vi "CRYLimits.vi"(0 "Setup in":T1={"No.VI"=0, "Category"="", "StepName"="", "Seq setup flattened"="", "Comment"="", "Steps config."=[], "Jump config"=[], "Start"=0.0, "Increment"=0.0, "Name"="Pa", "Unit"="Pa", "Y data"=1, "Y prefix"="", "Y dB ref"=1.0, "Y unit"="", "Repeat State Array"=[]} {"Repeat State Array"."Start" format="%#_5g"; "Y dB ref" format="%.1f"; "Y data" items=["dB", "Lin"]; "Start" format="%#_5g"}, 5 "Data in":T4 {"Z data" items=["dB", "Lin"]; "X data" items=["dB", "Lin"]; "Y data" items=["dB", "Lin"]; "Z dB ref" format="%.1f"; "Z axis" items=["Log", "Lin"]; "X dB ref" format="%.1f"; "X axis" items=["Log", "Lin"]; "Y axis" items=["Log", "Lin"]; "Y dB ref" format="%.1f"; "Curve"."z" format="%.2f"; "Curve"."y" format="%.2f"; "Curve"."x" format="%.2f"}, 7 "Results In":T2[](array[typedef]) {"Margin" format="%.2f"}, 9 "Seq setup in":string, 11 "Step Name":string, 12 "Hardware in":string, 13 "Calibration in":string) -> (3 "Types Out":string[](array[string]), 4 "Inserted Names Out":string[](array[string]), 6 "Data Out":T4 {"Z data" items=["dB", "Lin"]; "X data" items=["dB", "Lin"]; "Y data" items=["dB", "Lin"]; "Z dB ref" format="%.1f"; "Z axis" items=["Log", "Lin"]; "X dB ref" format="%.1f"; "X axis" items=["Log", "Lin"]; "Y axis" items=["Log", "Lin"]; "Y dB ref" format="%.1f"; "Curve"."z" format="%.2f"; "Curve"."y" format="%.2f"; "Curve"."x" format="%.2f"}, 8 "Results Out":T2[](array[typedef]) {"Margin" format="%.2f"}, 10 "Waveforms Out":T3[](array[typedef]) {"Y dB ref" format="%.1f"; "Y axis" items=["Log", "Lin"]; "Y data" items=["dB", "Lin"]; "X data" items=["dB", "Lin"]})   [LabVIEW 2013]
uses:
  Typedef Control/CRYData Cluster Array.ctl
  Typedef Control/CRYData Cluster.ctl
  Typedef Control/CRYWaveform Cluster.ctl
  Typedef Control/CRYResult Cluster.ctl
  Typedef Control/CRYStep.ctl
  <vilib>/event_ctls.llb/eventvkey.ctl
  Task Sequence/CRYProject Run Control Global.vi
  CRYStepSetup/CRYStepSetup Global.vi
  CRYLimit edit global.vi
  CRYMainGlobal.vi
panel:
  in  "Output failed":bool
  in  "Lim Curve axis lo":u16
  in  "Lim Curve axis up":u16
  out "Name":string
  in  "stop":bool
  in  "magn/phase":u16
  out "Multi unit":string="(und)"
  out "Multi Limit":cluster{dbl, dbl}(slide)={100.0, 4.285714285714286} caption="Upper limit" scale=-7.0..2.0 scale format="%.1p"
  out "Multi value":dbl(slide) scale=-7.0..2.0 scale format="%#.3p"
  in  "Lower Limit Type":u16
  in  "Upper Limit Type":u16
  in  "X-Resolution":u8
  in  "Data Selection Lower":u16
  in  "Data Selection Upper":u16
  in  "X axis":u16(slide)=1
  in  "Type":u16(slide)=1
  out "Limits Graph":cluster{"element":cluster{"x":dbl, "y":dbl}[]}[](graph)
  out "Limits Settings":bool
  in  "single val":bool
  in  "Data":cluster{"Hz":dbl, "dB":dbl}[](array[cluster])=[{"Hz"=1000.0, "dB"=125.0}] {"dB" format="%.1f"}
  in  "Tolerance":u16(ring)=2 caption="Alignment" items=["Individual Pts.", "Absolute Limits", "Floating Limits", "Floating Data", "Aligned Limits", "Aligned Data"]
  in  "Upper Limit":cluster{"Hz":dbl, "y":dbl}[](array[cluster])=[{"Hz"=1000.0, "y"=125.0}] {"y" format="%.1f"}
  in  "Lower Limit":cluster{"Hz":dbl, "y":dbl}[](array[cluster])=[{"Hz"=1000.0, "y"=125.0}] {"y" format="%.1f"}
  out "Data Out":cluster{dbl, dbl}[](array[cluster]) {"?" format="%.2f"; "?" format="%.2f"}
  out "Upper Limit Out":cluster{dbl, dbl}[](array[cluster]) {"?" format="%.2f"; "?" format="%.2f"}
  out "Lower Limit Out":cluster{dbl, dbl}[](array[cluster]) {"?" format="%.2f"; "?" format="%.2f"}
  in  "Align Reference":cluster{dbl, dbl}={1000.0, 0.0} {"?" format="%.1f"}
  out "Verdict":bool=TRUE
  out "Align Reference Out":cluster{dbl, dbl} {"?" format="%.2f"; "?" format="%.2f"}
  in  "Limits":u16(ring)=2 items=["Upper Only", "Lower Only", "Upper & Lower"]
  in  "Y-Resolution":u8
  out "max":dbl format="%.2f"
  out "min":dbl format="%.2f"
  out "y value":dbl format="%#.3p"
  out "Margin":dbl=-inf format="%_3p"
  in  "x float":bool caption="Float Limits in X"
  out "Unit":string
  out "Curve Name":string
  in  "Manual?":bool
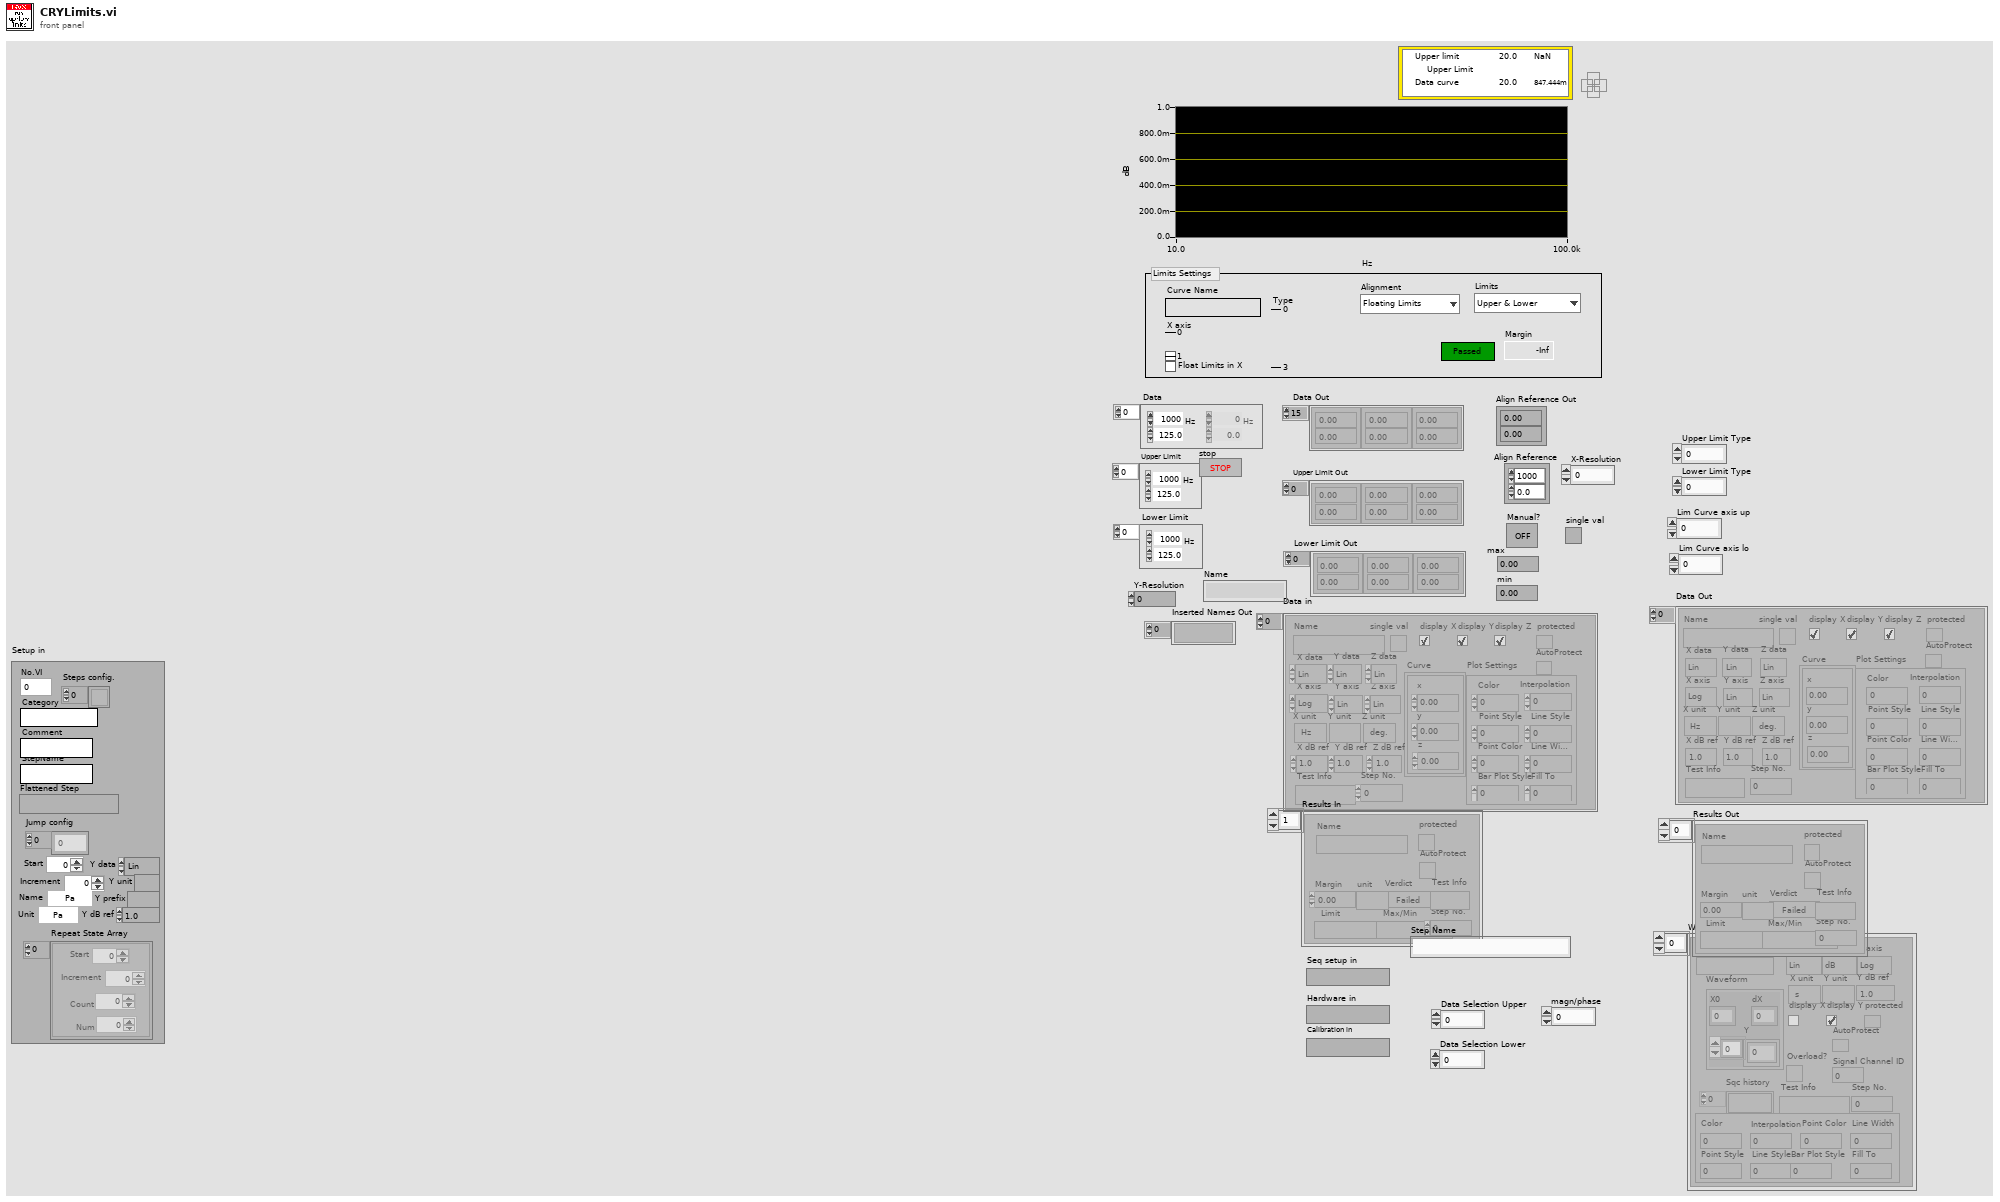
[diagram p1: front panel]
types:
  T1 = typedef "CRYStep.ctl" = cluster{"No.VI":i32, "Category":string, "StepName":string, "Seq setup flattened":string, "Comment":string, "Steps config.":bool[], "Jump config":i32[], "Start":dbl, "Increment":dbl, "Name":string, "Unit":string, "Y data":u16, "Y prefix":string, "Y dB ref":dbl, "Y unit":string, "Repeat State Array":cluster{"Start":dbl, "Increment":dbl, "Count":i32, "Num":i32}[]}
  T2 = typedef "CRYResult Cluster.ctl" = cluster{"Name":string, "Margin":dbl, "unit":string, "Verdict":bool, "Limit":string, "Max/Min":string, "protected":bool, "Step No.":i32, "Test Info":string, "AutoProtect":bool}
  T3 = typedef "CRYWaveform Cluster.ctl" = cluster{"Waveform":cluster{"X0":dbl, "dX":dbl, "Y":sgl[]}, "X data":u16, "Y data":u16, "Y axis":u16, "X unit":string, "Y unit":string, "Y dB ref":dbl, "display Y":bool, "display X":bool, "Overload?":bool, "Test Info":string, "Step No.":i32, "Name":string, "protected":bool, "Sqc history":string[], "Signal Channel ID":i32, "Plot Settings":cluster{"Color":u32, "Interpolation":u8, "Point Style":u8, "Line Style":u8, "Point Color":u32, "Line Width":u8, "Bar Plot Style":u8, "Fill To":i16}, "AutoProtect":bool}
  T4 = typedef "CRYData Cluster Array.ctl" = T5[]
  T5 = typedef "CRYData Cluster.ctl" = cluster{"Name":string, "Curve":cluster{"x":dbl, "y":dbl, "z":dbl}[], "X data":u16, "Y data":u16, "Z data":u16, "X axis":u16, "Y axis":u16, "Z axis":u16, "X unit":string, "Y unit":string, "Z unit":string, "X dB ref":dbl, "Y dB ref":dbl, "Z dB ref":dbl, "single val":bool, "protected":bool, "display X":bool, "display Y":bool, "display Z":bool, "Test Info":string, "Step No.":i32, "Plot Settings":cluster{"Color":u32, "Interpolation":u8, "Point Style":u8, "Line Style":u8, "Point Color":u32, "Line Width":u8, "Bar Plot Style":u8, "Fill To":i16}, "AutoProtect":bool}
  T6 = enum32{"Invalid", "Default", "Floating", "Floating/Auto-Hide", "Modal"}
  T7 = cluster{"Start":dbl, "Increment":dbl, "Count":i32, "Num":i32}[]
  T8 = typedef "CRYLimits.ctl" = cluster{"Name":string, "Tolerance":u16, "X Axis":u16, "Limits":u16, "Upper Limit":cluster{dbl, dbl}[], "Align Ref":cluster{dbl, dbl}, "Lower Limit":cluster{dbl, dbl}[], "Y data":u16, "Y unit":string, "Y dB ref":dbl, "Curve Names":string[], "Y-Resolution":u8, "Type":u16, "x float":bool, "X min-max-step":cluster{"Limit X Offset Min":dbl, "Limit X Offset Max":dbl, "Limit X Offset Step Size":dbl}, "magn/phase":u16, "Upper Limit Type":u16, "Lower Limit Type":u16, "Lim Curve axis up":u16, "Lim Curve axis lo":u16, "Data Selection Upper":u16, "Data Selection Lower":u16, "X-Resolution":u8, "Output failed point curves?":bool, "X data":u16, "X unit":string, "X dB ref":dbl, "X-Y Graph Set-up":string, "Tab Value":enum32{"Data", "Parameters"}, "Help":string, "X Up Val":dbl, "Y Up Val":dbl, "X Low Val":dbl, "Y Low Val":dbl, "Up Limit Val":dbl, "Low Limit Val":dbl, "bAdd DataName":bool, "Custom Name":string}
  T9 = cluster{"Limit X Offset Min":dbl, "Limit X Offset Max":dbl, "Limit X Offset Step Size":dbl}
  T10 = typedef "CRYWaveform Cluster Array.ctl" = T3[]
  T11 = enum32{"English", "Chinese", "Korean", "Japanese", "Russian", "Chinese traditional"}
  T12 = enum16{"OK", "Yes", "YesNo", "YesNoCancel", "ReplaceAppend"}
  T13 = cluster{"Lower Failed":cluster{"Hz":dbl, "y":dbl}[]}[]
  T14 = cluster{"Minimum":dbl, "Maximum":dbl, "Increment":dbl}
  T15 = typedef "eventvkey.ctl" = enum16{"ASCII", "Enter", "Return", "Shift", "Ctrl", "Alt", "Cmd", "Opt", "Caps", "NumLock", "Clear", "Break", "Up", "Down", "Left", "Right", "Insert", "Delete", "Home", "End", "PageUp", "PageDown", "Escape", "Help", "Pause", "ScrollLock", "F1", "F2", "F3", "F4", "F5", "F6", "F7", "F8", "F9", "F10", "F11", "F12", "F13", "F14", "F15", "F16", "F17", "F18", "F19", "F20", "F21", "F22", "F23", "F24", "Play", "VolumeUp", "VolumeDown", "Mute", "Two Byte Char"}
  T16 = typedef "CRYResult Cluster Array.ctl" = T2[]
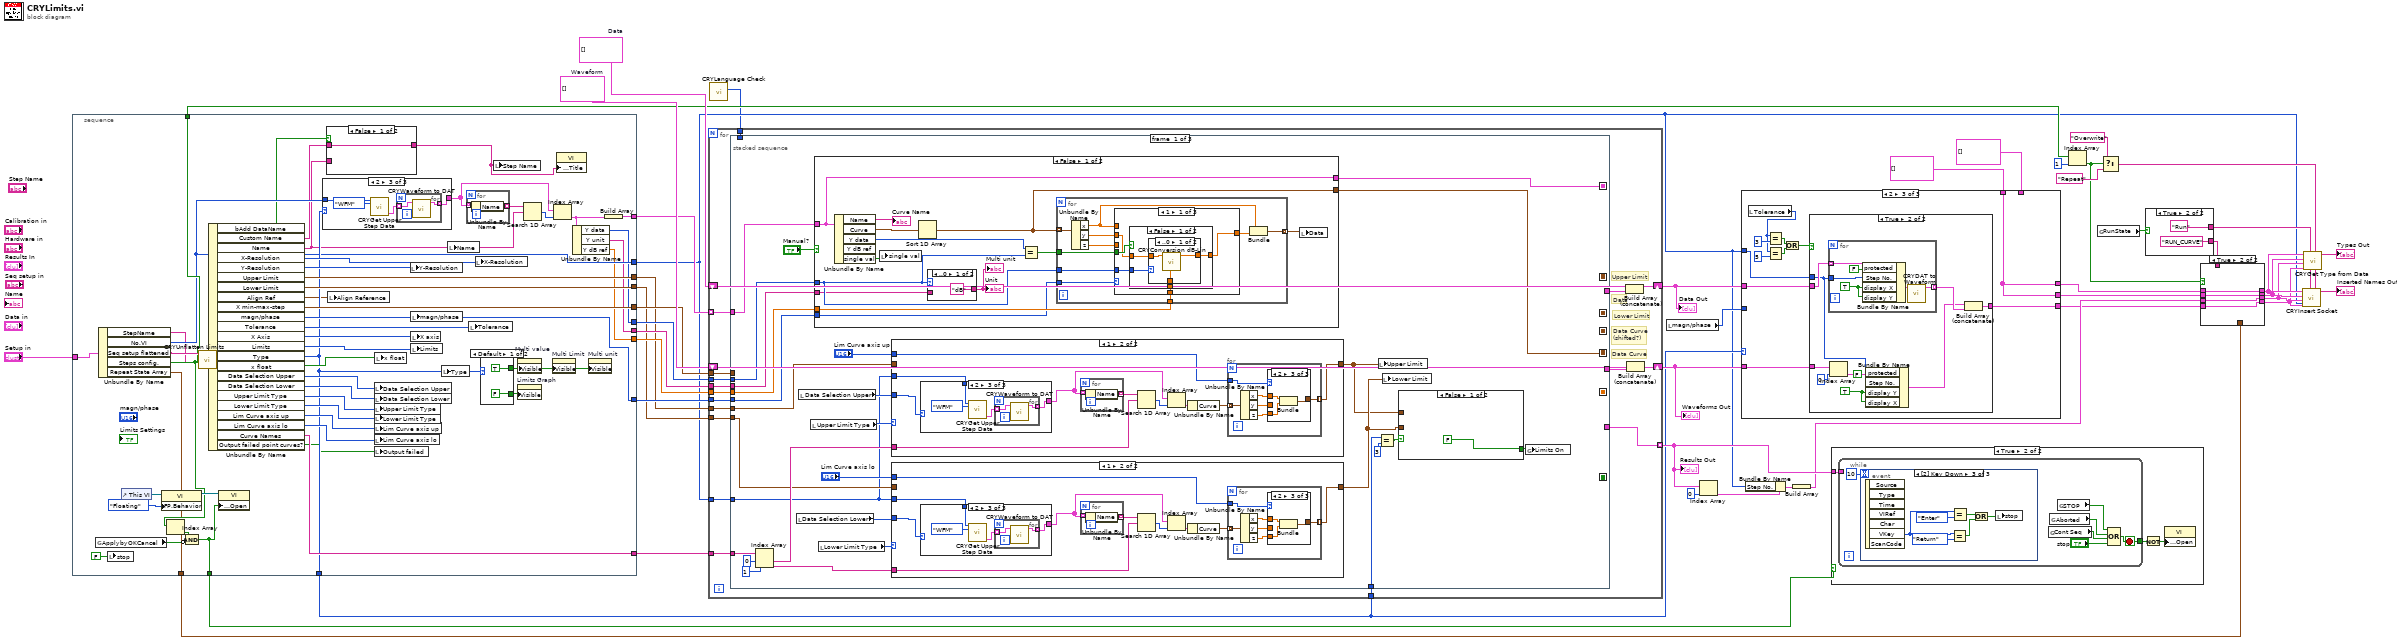
[diagram p0: block diagram]
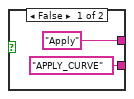
[diagram p2: hidden frame]
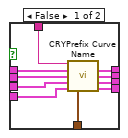
[diagram p3: hidden frame]
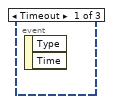
[diagram p5: hidden frame]
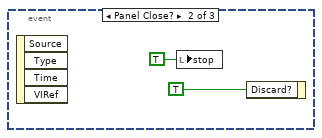
[diagram p6: hidden frame]
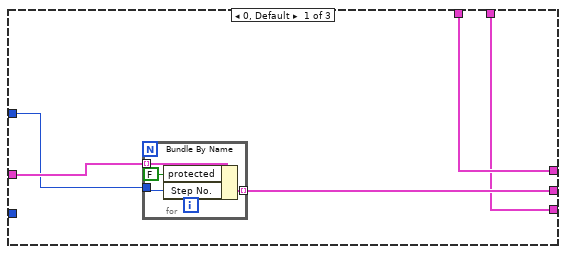
[diagram p7: hidden frame]
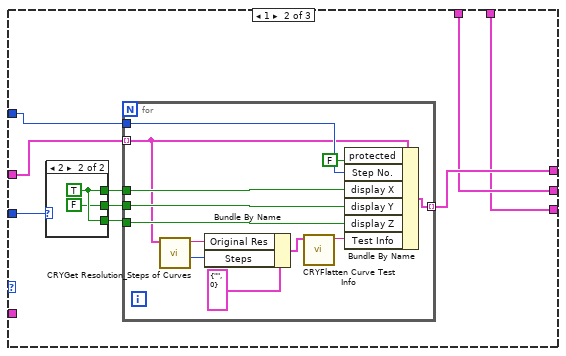
[diagram p8: hidden frame]
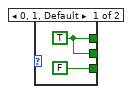
[diagram p9: hidden frame]
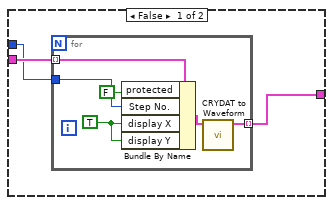
[diagram p10: hidden frame]
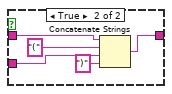
[diagram p11: hidden frame]
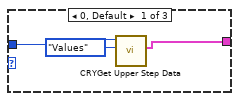
[diagram p12: hidden frame]
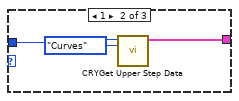
[diagram p13: hidden frame]
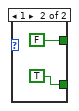
[diagram p14: hidden frame]
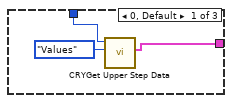
[diagram p16: hidden frame]
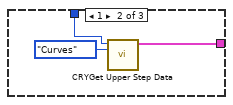
[diagram p17: hidden frame]
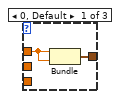
[diagram p18: hidden frame]
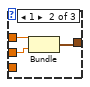
[diagram p19: hidden frame]
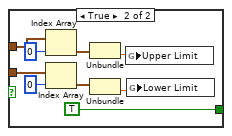
[diagram p20: hidden frame]
diagram:
  w44 = T3[] []  # Waveform
  w45 = T4 []  # Data
  n1 = stacked-sequence {
    tunnel: [w51] -> w43
    tunnel: [w52] -> w42
    tunnel: [w53] -> w41
    tunnel: [w82] -> w40
    tunnel: [w88] -> w27
    tunnel: [w65] -> w28
    tunnel: [w80] -> w34
    tunnel: [w55] -> w32
    tunnel: [w69] -> w31
    tunnel: [w68] -> w30
    tunnel: [w67] -> w29
    tunnel: [w59] -> w2
    tunnel: [w63] -> w20
    tunnel: [w62] -> w13
    tunnel: "Setup in" -> [w61]
    frame #0 {
      n2 = global read "CRYStepSetup Global.vi" "ApplybyOKCancel"() -> (w57:bool)
      n3 = Unbundle By Name(w61) -> ("StepName"=w46:string, "No.VI"=w59:i32, "Seq setup flattened"=w64:string, "Steps config."=w63:bool[], "Repeat State Array"=w62:T7)
      n4 = local write "stop"(FALSE ("stop")) -> ()
      n5 = control-ref of="This VI"() -> (w86:refnum<vi>)
      n6 = property class="VI"(reference=w86, "FP.Behavior"=T6."Floating" ("Front Panel Window:Behavior")) -> (reference out=w87:refnum<vi>)  [unwired: 1 in, 1 out]
      n7 = Index Array(array=w63) -> (element=w56:bool)  [unwired: 1 in]
      n8 = Compound Arithmetic op=AND(w56, invert w57) -> (w55:bool)
      n9 = call "CRYUnflatten Limits.vi"("Step Name"=w46, "Unflatten Limits"=w64) -> ("Limits"=w81:T8)  [unwired: 9 out]
      n10 = Unbundle By Name(w81) -> ("bAdd DataName"=w50:bool, "Custom Name"=w49:string, "Name"=w48:string, "X-Resolution"=w91:u8, "Y-Resolution"=w93:u8, "Upper Limit"=w69:cluster{dbl, dbl}[], "Lower Limit"=w68:cluster{dbl, dbl}[], "Align Ref"=w60:cluster{dbl, dbl}, "X min-max-step"=w82:T9, "magn/phase"=w80:u16, "Tolerance"=w79:u16, "X Axis"=w78:u16, "Limits"=w77:u16, "Type"=w65:u16, "x float"=w76:bool, "Data Selection Upper"=w75:u16, "Data Selection Lower"=w74:u16, "Upper Limit Type"=w73:u16, "Lower Limit Type"=w72:u16, "Lim Curve axis up"=w70:u16, "Lim Curve axis lo"=w71:u16, "Curve Names"=w67:string[], "Output failed point curves?"=w58:bool)
      n11 = property class="VI"(reference=w87, "Front Panel.Open"=w55) -> ()  [unwired: 1 in, 2 out]
      n12 = case shown="2" w65 {
        tunnel: w59 -> [w101 w104 w108]
        tunnel: [w100 w103 w106] -> w83
        frame 0, Default {
          n13 = call "CRYGet Upper Step Data.vi"("Type In"=enum16{"Curves", "Values", "Results", "WFM"}."Values" ("Type"), "No.VI"=w101) -> ("Value array"=w100:T4)  [unwired: 9 out]
        }
        frame 1 {
          n14 = call "CRYGet Upper Step Data.vi"("Type In"=enum16{"Curves", "Values", "Results", "WFM"}."Curves" ("Type"), "No.VI"=w104) -> ("Curve array"=w103:T4)  [unwired: 9 out]
        }
        frame 2 {
          n15 = call "CRYGet Upper Step Data.vi"("Type In"=enum16{"Curves", "Values", "Results", "WFM"}."WFM" ("Type"), "No.VI"=w108) -> ("Waveform Array"=w107:T10)  [unwired: 9 out]
          n16 = for {
            tunnel: [w111] -> w106 mode=indexing
            tunnel: w107 -> [w110] mode=indexing
            n17 = call "CRYWaveform to DAT.vi"("Waveform In"=w110) -> ("Curve Out"=w111:T5)  [unwired: 10 out]
          }
        }
      }
      n18 = case shown="False" w50 {
        tunnel: w49 -> [w94 w99]
        tunnel: w48 -> [_ w97]
        tunnel: [w94 w95] -> w47
        frame False {
        }
        frame True {
          n19 = Concatenate Strings(w99, "(" ("string"), w97, ")" ("string")) -> (w95:string)
        }
      }
      n20 = local write "Align Reference"(w60) -> ()
      n21 = local write "Data Selection Upper"(w75) -> ()
      n22 = local write "Data Selection Lower"(w74) -> ()
      n23 = local write "Upper Limit Type"(w73) -> ()
      n24 = local write "Lower Limit Type"(w72) -> ()
      n25 = local write "Lim Curve axis up"(w70) -> ()
      n26 = local write "Lim Curve axis lo"(w71) -> ()
      n27 = local write "Output failed"(w58) -> ()
      n28 = local write "x float"(w76) -> ()
      n29 = local write "Y-Resolution"(w93) -> ()
      n30 = local write "magn/phase"(w80) -> ()
      n31 = local write "X axis"(w78) -> ()
      n32 = local write "Limits"(w77) -> ()
      n33 = local write "Type"(w65) -> ()
      n34 = local write "Name"(w48) -> ()
      n35 = for {
        tunnel: w83 -> [w113] mode=indexing
        tunnel: [w112] -> w90 mode=indexing
        n36 = Unbundle By Name(w113) -> ("Name"=w112:string)
      }
      n37 = local write "Tolerance"(w79) -> ()
      n38 = local write "X-Resolution"(w91) -> ()
      n39 = case shown="Default" w65 {
        tunnel: [TRUE FALSE] -> w92
        tunnel: [FALSE TRUE] -> w66
        frame Default {
        }
        frame 1 {
        }
      }
      n40 = local write "Step Name"(w47) -> ()
      n41 = property on="Limits Graph" class="XYGraph (strict)"("Visible"=w66) -> ()  [unwired: 2 in, 2 out]
      n42 = property on="Multi value" class="Slide (strict)"("Visible"=w92) -> ()  [unwired: 2 in, 2 out]
      n43 = Search 1D Array(1D array=w90, element=w48) -> (index of element=w89:i32)  [unwired: 1 in]
      n44 = property on="Multi Limit" class="Slide (strict)"("Visible"=w92) -> ()  [unwired: 2 in, 2 out]
      n45 = Index Array(array=w83, index=w89) -> (element=w54:T5)
      n46 = property class="VI"("Front Panel.Title"=w47) -> ()  [unwired: 2 in, 2 out]
      n47 = Unbundle By Name(w54) -> ("Y data"=w53:u16, "Y unit"=w52:string, "Y dB ref"=w51:dbl)
      n48 = property on="Multi unit" class="Str"("Visible"=w92) -> ()  [unwired: 2 in, 2 out]
      n49 = Build Array(w54) -> (w88:T5[])
    }
  }
  n50 = call "CRYLanguage Check.vi"() -> ("Language"=w1:T11)  [unwired: 10 in, 1 out]
  n51 = for {
    tunnel: w43 -> [w136]
    tunnel: w42 -> [w135]
    tunnel: w41 -> [w134]
    tunnel: [w133] -> w33 mode=indexing
    tunnel: w27 -> [w132] mode=indexing
    shift-right: [w130] -> w37
    shift-left: w45 -> [w129]
    tunnel: w40 -> [w128]
    tunnel: w34 -> [w127]
    shift-right: [w126] -> w39
    shift-left: w44 -> [w125]
    tunnel: w31 -> [w123]
    tunnel: w30 -> [w122]
    tunnel: w29 -> [w121]
    tunnel: w28 -> [w120]
    tunnel: w2 -> [w119]
    tunnel: w1 -> [w118]
    # "Data Curve\n(shifted?)"
    # "Lower Limit"
    # "Upper Limit"
    # "Data"
    # "Data Curve"
    n52 = stacked-sequence {
      seq-local: [_ w330 _] -> [_ _ w574]
      seq-local: [_ w329 _] -> [_ _ w570]
      seq-local: [_ w331 _] -> [_ _ w568]
      seq-local: [w164 _ _] -> [_ _ w567]
      seq-local: [w163 _ _] -> [_ _ w536]
      seq-local: [_ w339 _] -> [_ _ w532]
      seq-local: [_ w338 _] -> [_ _ w537]
      tunnel: w134 -> [w162 _ w552]
      tunnel: w135 -> [w160 _ _]
      tunnel: w136 -> [w161 _ w560]
      tunnel: [_ _ w549] -> w133
      tunnel: [_ _ w559] -> w131
      tunnel: w132 -> [w159 _ w539]
      tunnel: w128 -> [_ w333 _]
      tunnel: w127 -> [w157 _ w533]
      tunnel: [_ _ w541] -> w124
      tunnel: w123 -> [w153 _ _]
      tunnel: w122 -> [w143 _ _]
      tunnel: w121 -> [w151 _ _]
      tunnel: w120 -> [w139 _ _]
      tunnel: w119 -> [w137 _ _]
      tunnel: w118 -> [_ _ w519]
      frame #0 {
        n53 = Index Array(array=w151, index #1=0 ("index"), index #2=1 ("index")) -> (element #1=w149:string, element #2=w146:string)
        n54 = local read "Data Selection Lower"() -> (w142:u16)
        n55 = local read "Data Selection Upper"() -> (w152:u16)
        n56 = local read "Upper Limit Type"() -> (w156:u16)
        n57 = case shown="False" "Manual?" {
          tunnel: w159 -> [w258 _]
          tunnel: w160 -> [w257 _]
          tunnel: w161 -> [w265 _]
          tunnel: w162 -> [w264 _]
          tunnel: [w258 w297] -> w163
          tunnel: [w254 cluster{"x":dbl, "y":dbl, "z":dbl}[] [] ("Curve")] -> w164
          tunnel: w157 -> [w256 _]
          frame False {
            n58 = Unbundle By Name(w258) -> ("Name"=→"Curve Name":string, "Curve"=w261:cluster{"x":dbl, "y":dbl, "z":dbl}[], "Y data"=w263:u16, "single val"=w259:bool)  [unwired: 1 out]
            n59 = local write "single val"(w259) -> ()
            n60 = Sort 1D Array(array=w261) -> (sorted array=w254:cluster{"x":dbl, "y":dbl, "z":dbl}[])
            n61 = case shown="..0" w264 {
              tunnel: ["dB" w295] -> w255
              tunnel: w257 -> [_ w295]
              frame ..0 {
              }
              frame 1.. {
              }
            }
            "Unit" <- w255
            "Multi unit" <- w255
            n62 = Equal?(x=w263, y=w264) -> (x = y?=w262:bool)
            n63 = for {
              tunnel: w254 -> [w275] mode=indexing
              tunnel: [w273] -> w253 mode=indexing
              tunnel: w262 -> [w272]
              tunnel: w265 -> [w271]
              tunnel: w264 -> [w270]
              tunnel: w256 -> [w268]
              n64 = Unbundle By Name(w275) -> ("x"=w274:dbl, "y"=w267:dbl, "z"=w269:dbl)
              n65 = case shown="1" w268 {
                tunnel: w270 -> [w280 _ _]
                tunnel: w271 -> [w279 _ _]
                tunnel: w272 -> [w278 _ _]
                tunnel: w267 -> [w277 _ _]
                tunnel: [w276 w292 w293] -> w266
                tunnel: w269 -> [_ w292 _]
                tunnel: w274 -> [_ _ w293]
                frame 1 {
                  n66 = case shown="False" w278 {
                    tunnel: [w284 w291] -> w276
                    tunnel: w277 -> [w283 w291]
                    tunnel: w279 -> [w282 _]
                    tunnel: w280 -> [w281 _]
                    frame False {
                      n67 = case shown="..0" w281 {
                        tunnel: w282 -> [w287 w289]
                        tunnel: w283 -> [w285 w290]
                        tunnel: [w286 w288] -> w284
                        frame ..0 {
                          n68 = call "CRYConversion dB-Lin.vi"("dB ref."=w287, "Lin In"=w285) -> ("Log Out"=w286:dbl)  [unwired: 4 in, 3 out]
                        }
                        frame 1.. {
                          n69 = call "CRYConversion dB-Lin.vi"("dB ref."=w289, "Log In"=w290) -> ("Lin Out"=w288:dbl)  [unwired: 4 in, 3 out]
                        }
                      }
                    }
                    frame True {
                    }
                  }
                }
                frame 2 {
                }
                frame 0, Default {
                }
              }
              n70 = Bundle("x"=w274, "x"=w266) -> (w273:cluster{"x":dbl, "x":dbl})  [unwired: 1 out]
            }
            n71 = local write "Data"(w253) -> ()
          }
          frame True {
            n72 = local write "single val"(FALSE ("single val")) -> ()
            n73 = call "CRYUnflatten Data.vi"() -> ("Datum"=w297:T5)  [unwired: 1 in, 10 out]
          }
        }
        n74 = local read "Lower Limit Type"() -> (w144:u16)
        n75 = case shown="1" w156 {
          tunnel: w153 -> [w214 _]
          tunnel: [w214 w215] -> w140
          tunnel: w152 -> [_ w223]
          tunnel: w137 -> [_ w224]
          tunnel: w149 -> [_ w219]
          tunnel: "Lim Curve axis up" -> [_ w216]
          frame 0, Default {
          }
          frame 1 {
            n76 = case shown="2" w223 {
              tunnel: w224 -> [w226 w229 w233]
              tunnel: [w225 w228 w231] -> w220
              frame 0, Default {
                n77 = call "CRYGet Upper Step Data.vi"("Type In"=enum16{"Curves", "Values", "Results", "WFM"}."Values" ("Type"), "No.VI"=w226) -> ("Value array"=w225:T4)  [unwired: 9 out]
              }
              frame 1 {
                n78 = call "CRYGet Upper Step Data.vi"("Type In"=enum16{"Curves", "Values", "Results", "WFM"}."Curves" ("Type"), "No.VI"=w229) -> ("Curve array"=w228:T4)  [unwired: 9 out]
              }
              frame 2 {
                n79 = call "CRYGet Upper Step Data.vi"("Type In"=enum16{"Curves", "Values", "Results", "WFM"}."WFM" ("Type"), "No.VI"=w233) -> ("Waveform Array"=w232:T10)  [unwired: 9 out]
                n80 = for {
                  tunnel: [w236] -> w231 mode=indexing
                  tunnel: w232 -> [w235] mode=indexing
                  n81 = call "CRYWaveform to DAT.vi"("Waveform In"=w235) -> ("Curve Out"=w236:T5)  [unwired: 10 out]
                }
              }
            }
            n82 = for {
              tunnel: w220 -> [w252] mode=indexing
              tunnel: [w251] -> w222 mode=indexing
              n83 = Unbundle By Name(w252) -> ("Name"=w251:string)
            }
            n84 = Search 1D Array(1D array=w222, element=w219) -> (index of element=w221:i32)  [unwired: 1 in]
            n85 = Index Array(array=w220, index=w221) -> (element=w218:T5)
            n86 = Unbundle By Name(w218) -> ("Curve"=w217:cluster{"x":dbl, "y":dbl, "z":dbl}[])
            n87 = for {
              tunnel: w217 -> [w242] mode=indexing
              tunnel: w216 -> [w241]
              tunnel: [w237] -> w215 mode=indexing
              n88 = Unbundle By Name(w242) -> ("x"=w240:dbl, "y"=w239:dbl, "z"=w238:dbl)
              n89 = case shown="2" w241 {
                tunnel: w240 -> [w244 w247 w249]
                tunnel: w239 -> [_ w246 _]
                tunnel: w238 -> [_ _ w250]
                tunnel: [w243 w245 w248] -> w237
                frame 0, Default {
                  n90 = Bundle("x"=w244, "x"=w244) -> (w243:cluster{"x":dbl, "x":dbl})  [unwired: 1 in]
                }
                frame 1 {
                  n91 = Bundle("x"=w247, "y"=w246) -> (w245:cluster{"x":dbl, "y":dbl})  [unwired: 1 in]
                }
                frame 2 {
                  n92 = Bundle("x"=w249, "z"=w250) -> (w248:cluster{"x":dbl, "z":dbl})  [unwired: 1 in]
                }
              }
            }
          }
        }
        n93 = case shown="1" w144 {
          tunnel: w143 -> [w165 _]
          tunnel: [w165 w166] -> w141
          tunnel: w142 -> [_ w174]
          tunnel: w137 -> [_ w175]
          tunnel: w146 -> [_ w170]
          tunnel: "Lim Curve axis lo" -> [_ w167]
          frame 0, Default {
          }
          frame 1 {
            n94 = case shown="2" w174 {
              tunnel: w175 -> [w177 w180 w184]
              tunnel: [w176 w179 w182] -> w171
              frame 0, Default {
                n95 = call "CRYGet Upper Step Data.vi"("Type In"=enum16{"Curves", "Values", "Results", "WFM"}."Values" ("Type"), "No.VI"=w177) -> ("Value array"=w176:T4)  [unwired: 9 out]
              }
              frame 1 {
                n96 = call "CRYGet Upper Step Data.vi"("Type In"=enum16{"Curves", "Values", "Results", "WFM"}."Curves" ("Type"), "No.VI"=w180) -> ("Curve array"=w179:T4)  [unwired: 9 out]
              }
              frame 2 {
                n97 = call "CRYGet Upper Step Data.vi"("Type In"=enum16{"Curves", "Values", "Results", "WFM"}."WFM" ("Type"), "No.VI"=w184) -> ("Waveform Array"=w183:T10)  [unwired: 9 out]
                n98 = for {
                  tunnel: [w187] -> w182 mode=indexing
                  tunnel: w183 -> [w186] mode=indexing
                  n99 = call "CRYWaveform to DAT.vi"("Waveform In"=w186) -> ("Curve Out"=w187:T5)  [unwired: 10 out]
                }
              }
            }
            n100 = for {
              tunnel: w171 -> [w203] mode=indexing
              tunnel: [w202] -> w173 mode=indexing
              n101 = Unbundle By Name(w203) -> ("Name"=w202:string)
            }
            n102 = Search 1D Array(1D array=w173, element=w170) -> (index of element=w172:i32)  [unwired: 1 in]
            n103 = Index Array(array=w171, index=w172) -> (element=w169:T5)
            n104 = Unbundle By Name(w169) -> ("Curve"=w168:cluster{"x":dbl, "y":dbl, "z":dbl}[])
            n105 = for {
              tunnel: w168 -> [w193] mode=indexing
              tunnel: w167 -> [w192]
              tunnel: [w188] -> w166 mode=indexing
              n106 = Unbundle By Name(w193) -> ("x"=w191:dbl, "y"=w190:dbl, "z"=w189:dbl)
              n107 = case shown="2" w192 {
                tunnel: w191 -> [w195 w198 w200]
                tunnel: w190 -> [_ w197 _]
                tunnel: w189 -> [_ _ w201]
                tunnel: [w194 w196 w199] -> w188
                frame 0, Default {
                  n108 = Bundle("x"=w195, "x"=w195) -> (w194:cluster{"x":dbl, "x":dbl})  [unwired: 1 in]
                }
                frame 1 {
                  n109 = Bundle("x"=w198, "y"=w197) -> (w196:cluster{"x":dbl, "y":dbl})  [unwired: 1 in]
                }
                frame 2 {
                  n110 = Bundle("x"=w200, "z"=w201) -> (w199:cluster{"x":dbl, "z":dbl})  [unwired: 1 in]
                }
              }
            }
          }
        }
        n111 = local write "Upper Limit"(w140) -> ()
        n112 = Equal?(x=w139, y=u16 3) -> (x = y?=w155:bool)
        n113 = local write "Lower Limit"(w141) -> ()
        n114 = case shown="False" w155 {
          tunnel: [FALSE ("Limits On") TRUE ("Limits On")] -> w154
          tunnel: w140 -> [_ w212]
          tunnel: w141 -> [_ w211]
          frame False {
          }
          frame True {
            n115 = Index Array(array=w212, index=0) -> (element=w208:cluster{"x":dbl, "z":dbl})
            n116 = Index Array(array=w211, index=0) -> (element=w207:cluster{"x":dbl, "z":dbl})
            n117 = Unbundle(w208) -> ("z"=w206:dbl)  [unwired: 1 out]
            n118 = Unbundle(w207) -> ("z"=w205:dbl)  [unwired: 1 out]
            n119 = global write "CRYLimit edit global.vi" "Upper Limit"(w206) -> ()
            n120 = global write "CRYLimit edit global.vi" "Lower Limit"(w205) -> ()
          }
        }
        n121 = global write "CRYLimit edit global.vi" "Limits On"(w154) -> ()
      }
      frame #1 {
        n122 = Sort 1D Array(array="Data") -> (sorted array=w332:cluster{"Hz":dbl, "dB":dbl}[])
        n123 = Equal?(x=u16 1, y="Upper Limit Type") -> (x = y?=w318:bool)
        n124 = Equal To 0?(x="Data Selection Upper") -> (x = 0?=w319:bool)
        n125 = And(x=w318, y=w319) -> (x .and. y?=w311:bool)
        n126 = Equal To 0?(x="Data Selection Lower") -> (x = 0?=w313:bool)
        n127 = Equal?(x="Lower Limit Type", y=u16 1) -> (x = y?=w312:bool)
        n128 = And(x=w313, y=w312) -> (x .and. y?=w314:bool)
        n129 = case shown="0, Default" "X axis" {
          tunnel: "Upper Limit" -> [w369 w374]
          tunnel: [w366 w370] -> w306
          frame 0, Default {
            n130 = Array Size(array=w369) -> (size(s)=w368:i32)
            n131 = Equal?(x=w368, y=1) -> (x = y?=w366:bool)
          }
          frame 1 {
            n132 = for {
              tunnel: w374 -> [w387] mode=indexing
              tunnel: [w386] -> w375 mode=indexing
              n133 = Unbundle(w387) -> ("Hz"=w386:dbl)  [unwired: 1 out]
            }
            n134 = for {
              shift-right: [w380] -> w373
              shift-left: w374 -> [w381]
              tunnel: w375 -> [w379] mode=indexing
              i -> [w376]
              n135 = Less?(x=w379, y=0.0) -> (x < y?=w377:bool)
              n136 = case shown="False" w377 {
                tunnel: w381 -> [w382 w385]
                tunnel: [w382 w384] -> w380
                tunnel: w376 -> [_ w383]
                frame False {
                }
                frame True {
                  n137 = Delete From Array(array=w385, index=w383) -> (array with subset deleted=w384:cluster{"Hz":dbl, "y":dbl}[])  [unwired: 1 in, 1 out]
                }
              }
            }
            n138 = Array Size(array=w373) -> (size(s)=w372:i32)
            n139 = Equal?(x=w372, y=1) -> (x = y?=w370:bool)
          }
        }
        n140 = case shown="1" "X axis" {
          tunnel: "Lower Limit" -> [w347 w352]
          tunnel: [w344 w348] -> w305
          frame 0, Default {
            n141 = Array Size(array=w347) -> (size(s)=w346:i32)
            n142 = Equal?(x=w346, y=1) -> (x = y?=w344:bool)
          }
          frame 1 {
            n143 = for {
              tunnel: w352 -> [w365] mode=indexing
              tunnel: [w364] -> w353 mode=indexing
              n144 = Unbundle(w365) -> ("Hz"=w364:dbl)  [unwired: 1 out]
            }
            n145 = for {
              shift-right: [w358] -> w351
              shift-left: w352 -> [w359]
              tunnel: w353 -> [w357] mode=indexing
              i -> [w354]
              n146 = Less?(x=w357, y=0.0) -> (x < y?=w355:bool)
              n147 = case shown="True" w355 {
                tunnel: w359 -> [w360 w363]
                tunnel: [w360 w362] -> w358
                tunnel: w354 -> [_ w361]
                frame False {
                }
                frame True {
                  n148 = Delete From Array(array=w363, index=w361) -> (array with subset deleted=w362:cluster{"Hz":dbl, "y":dbl}[])  [unwired: 1 in, 1 out]
                }
              }
            }
            n149 = Array Size(array=w351) -> (size(s)=w350:i32)
            n150 = Equal?(x=w350, y=1) -> (x = y?=w348:bool)
          }
        }
        n151 = Compound Arithmetic op=OR(w311, w314, w306, w305) -> (w303:bool)
        n152 = case shown="False" w303 {
          tunnel: ["Tolerance" u16 0 ("Tolerance")] -> w310
          frame False {
          }
          frame True {
          }
        }
        n153 = case shown="0, Default" "Type" {
          tunnel: [w393 w432 w446] -> w341
          tunnel: "Align Reference" -> [w393 w433 w458]
          tunnel: "X axis" -> [_ w437 _]
          tunnel: "Lower Limit" -> [w409 w425 w443]
          tunnel: "Upper Limit" -> [w410 w426 w445]
          tunnel: w310 -> [_ w424 w440]
          tunnel: [w403 w430 w448] -> w330
          tunnel: [w401 w431 w447] -> w329
          tunnel: [w397 w422 w451] -> w339
          tunnel: [w394 w428 w450] -> w338
          tunnel: [TRUE ("Visible") FALSE ("Visible") FALSE ("Visible")] -> w304
          tunnel: "Limits" -> [w412 w434 w459]
          tunnel: w332 -> [w400 w423 w460]
          tunnel: [w399 w429 w449] -> w331
          tunnel: [w396 w422 w451] -> w336
          tunnel: "x float" -> [_ w438 w454]
          tunnel: "Y-Resolution" -> [w390 w421 w457]
          tunnel: w333 -> [_ w427 w456]
          tunnel: "Data Selection Upper" -> [_ _ w444]
          tunnel: "Data Selection Lower" -> [_ _ w442]
          frame 0, Default {
            # "Single Value"
            n154 = Index Array(array=w410, index=0) -> (element=w404:cluster{"Hz":dbl, "y":dbl})
            n155 = Index Array(array=w409, index=0) -> (element=w402:cluster{"Hz":dbl, "y":dbl})
            n156 = Index Array(array=w400, index=0) -> (element=w398:cluster{"Hz":dbl, "dB":dbl})
            n157 = Unbundle(w404) -> ("y"=w405:dbl)  [unwired: 1 out]
            n158 = Unbundle(w398) -> ("dB"=w397:dbl)  [unwired: 1 out]
            "y value" <- w397
            n159 = Unbundle(w402) -> ("y"=w406:dbl)  [unwired: 1 out]
            n160 = case shown="Default" w412 {
              tunnel: [w415 w416 inf ("y")] -> w392
              tunnel: [w414 -inf ("y") w418] -> w391
              tunnel: w405 -> [w415 w416 _]
              tunnel: w406 -> [w414 _ w418]
              frame Default {
              }
              frame 0 {
              }
              frame 1 {
              }
            }
            "max" <- w392
            "min" <- w391
            n161 = Build Array(w404) -> (w403:cluster{"Hz":dbl, "y":dbl}[])
            n162 = Build Array(w402) -> (w401:cluster{"Hz":dbl, "y":dbl}[])
            n163 = Build Array(w398) -> (w399:cluster{"Hz":dbl, "dB":dbl}[])
            n164 = call "CRYRepresent numeric by precission.vi"("Pprecision"=w390, "Numeric In"=w392) -> ("Numeric Out"=w389:dbl)  [unwired: 7 in, 2 out]
            n165 = call "CRYRepresent numeric by precission.vi"("Pprecision"=w390, "Numeric In"=w391) -> ("Numeric Out"=w388:dbl)  [unwired: 7 in, 2 out]
            n166 = call "CRYRepresent numeric by precission.vi"("Pprecision"=w390, "Numeric In"=w397) -> ("Out Format"=w395:string, "Numeric Out"=w396:dbl)  [unwired: 7 in, 1 out]
            n167 = property on="Margin" class="DigNum (strict)"("FormatString"=w395) -> ()  [unwired: 2 in, 2 out]
            n168 = In Range and Coerce(upper limit=w389, x=w396, lower limit=w388) -> (In Range?=w394:bool)  [unwired: 1 out]
          }
          frame 1 {
            # "Curve"
            n169 = Boolean To (0,1)(Boolean=w438) -> (0, 1=w436:i16)
            n170 = To Unsigned Word Integer(number=w436) -> (unsigned 16bit integer=w435:u16)
            n171 = call "CRYMR_TOL2.vi"("Tolerance"=w424, "X Floating Limits"=w435, "x axis"=w437, "Limits"=w434, "X min-max-step"=w427, "Data"=w423, "Upper Limit"=w426, "Lower Limit"=w425, "Align Reference"=w433, "Resolution (decimals)"=w421) -> ("Margin"=w422:dbl, "Verdict"=w428:bool, "Data Out"=w429:cluster{dbl, dbl}[], "Upper Limit Out"=w430:cluster{dbl, dbl}[], "Align Reference Out"=w432:cluster{dbl, dbl}, "Lower Limit Out"=w431:cluster{dbl, dbl}[])
            n172 = call "CRYRepresent numeric by precission.vi"("Pprecision"=w421, "Numeric In"=w422) -> ("Out Format"=w420:string)  [unwired: 7 in, 2 out]
            n173 = property on="Margin" class="DigNum (strict)"("FormatString"=w420) -> ()  [unwired: 2 in, 2 out]
          }
          frame 2 {
            w464 = u16 2 ("y")
            # "Waveform"
            n174 = Not Equal?(x=w444, y=w464) -> (x != y?=w463:bool)
            n175 = Not Equal?(x=w464, y=w442) -> (x != y?=w462:bool)
            n176 = And(x=w463, y=w462) -> (x .and. y?=w461:bool)
            n177 = Boolean To (0,1)(Boolean=w454) -> (0, 1=w455:i16)
            n178 = To Unsigned Word Integer(number=w455) -> (unsigned 16bit integer=w453:u16)
            n179 = case shown="True" w461 {
              tunnel: w460 -> [w474 w493]
              tunnel: w445 -> [w476 w492]
              tunnel: w443 -> [w475 w491]
              tunnel: u16 0 ("X axis") -> [_ w490]
              tunnel: w440 -> [_ w489]
              tunnel: w459 -> [_ w488]
              tunnel: w458 -> [w473 w487]
              tunnel: w457 -> [_ w477]
              tunnel: w456 -> [_ w486]
              tunnel: w453 -> [_ w485]
              tunnel: [inf w478] -> w451
              tunnel: [FALSE ("Verdict") w484] -> w450
              tunnel: [w474 w483] -> w449
              tunnel: [w476 w482] -> w448
              tunnel: [w475 w481] -> w447
              tunnel: [w473 w480] -> w446
              frame False {
                w470 = cluster{dbl, dbl}[] [] ("critical point")
                n180 = call "CRYGet Error Message.vi"("Error No"=1, "Kind"="Limits") -> ("Message"=w467:string, "Window Title"=w466:string)  [unwired: 4 in, 4 out]
                n181 = global write "CRYLimit edit global.vi" "critical point"(w470) -> ()
                n182 = global write "CRYLimit edit global.vi" "align ref point"(w470) -> ()
                n183 = global write "CRYLimit edit global.vi" "Upper Failed"(w470) -> ()
                n184 = global write "CRYLimit edit global.vi" "Lower Failed"(w470) -> ()
                n185 = call "CRYMessage Dialog.vi"("Window Title"=w466, "YesNoCancel"=T12."OK", "Message Content"=w467) -> ()  [unwired: 7 in, 2 out]
              }
              frame True {
                n186 = call "CRYMR_TOL2.vi"("Tolerance"=w489, "X Floating Limits"=w485, "x axis"=w490, "Limits"=w488, "X min-max-step"=w486, "Data"=w493, "Upper Limit"=w492, "Lower Limit"=w491, "Align Reference"=w487, "Resolution (decimals)"=w477) -> ("Margin"=w478:dbl, "Verdict"=w484:bool, "Data Out"=w483:cluster{dbl, dbl}[], "Upper Limit Out"=w482:cluster{dbl, dbl}[], "Align Reference Out"=w480:cluster{dbl, dbl}, "Lower Limit Out"=w481:cluster{dbl, dbl}[])
                n187 = call "CRYRepresent numeric by precission.vi"("Pprecision"=w477, "Numeric In"=w478) -> ("Out Format"=w479:string)  [unwired: 7 in, 2 out]
                n188 = property on="Margin" class="DigNum (strict)"("FormatString"=w479) -> ()  [unwired: 2 in, 2 out]
              }
            }
          }
        }
        "Data Out" <- w331
        "Upper Limit Out" <- w330
        "Lower Limit Out" <- w329
        "Verdict" <- w338
        "Align Reference Out" <- w341
        "Margin" <- w336
        n189 = property on="y value" class="DigNum (strict)"("Visible"=w304) -> ()  [unwired: 2 in, 2 out]
        n190 = stacked-sequence {
          tunnel: w331 -> [_]
          tunnel: [w497] -> w328
          tunnel: [w496] -> w327
          tunnel: [w495] -> w326
          tunnel: [w494] -> w325
          frame #0 {
            n191 = global read "CRYLimit edit global.vi" "align ref point"() -> (w496:cluster{dbl, dbl}[])
            n192 = global read "CRYLimit edit global.vi" "critical point"() -> (w497:cluster{dbl, dbl}[])
            n193 = global read "CRYLimit edit global.vi" "Upper Failed"() -> (w495:cluster{dbl, dbl}[])
            n194 = global read "CRYLimit edit global.vi" "Lower Failed"() -> (w494:cluster{dbl, dbl}[])
          }
        }
        n195 = Build Cluster Array(w331, w330, w329, w328, w327, w326, w325) -> (w302:T13)
        n196 = local read "X-Resolution"() -> (w301:u8)
        n197 = local read "Y-Resolution"() -> (w300:u8)
        n198 = case shown="1, 2" "Type" {
          tunnel: w302 -> [w501 w507]
          tunnel: w301 -> [_ w503]
          tunnel: w300 -> [_ w502]
          frame 0, Default {
            n199 = call "CRYSingle Limit bar.vi"("Limit Graph"=w501) -> ("Scale range info"=w500:T14, "Limits bar"=→"Multi Limit":cluster{dbl, dbl}, "Single value"=→"Multi value":dbl)  [unwired: 8 out]
            n200 = property on="Multi value" class="Slide (strict)"("Scale.Old Range"=w500) -> ()  [unwired: 2 in, 2 out]
            n201 = property on="Multi Limit" class="Slide (strict)"("Scale.Old Range"=w500) -> ()  [unwired: 2 in, 2 out]
          }
          frame 1, 2 {
            n202 = local read "Tolerance"() -> (w505:u16)
            n203 = local read "Limits"() -> (w504:u16)
            n204 = stacked-sequence {
              seq-local: [w514 _ _ _] -> [_ _ _ w516]
              tunnel: w507 -> [w513 w515 _ _]
              tunnel: "Output failed" -> [w512 _ _ _]
              tunnel: w505 -> [w511 _ _ _]
              tunnel: w504 -> [w510 _ _ _]
              tunnel: w503 -> [w509 _ _ _]
              tunnel: w502 -> [w508 _ _ _]
              frame #0 {
                n205 = control-ref of="Limits Graph"() -> (w514:refnum<vi>)
                n206 = call "CRYGet Max Min from XY Graph Data.vi"("Limits"=w510, "Limits Graph"=w514, "Output failed"=w512, "X-Resolution"=w509, "Y-Resolution"=w508, "Tolerance"=w511, "array of clusters"=w513) -> ()  [unwired: 9 in]
              }
              frame #1 {
                "Limits Graph" <- w515
              }
              frame #2 {
              }
              frame #3 {
                n207 = call "CRYPaint WaterMark.vi"("Type"="Small", "Graph Ref"=w516) -> ()  [unwired: 10 in]
              }
            }
          }
        }
        n208 = property on="Limits Graph" class="XYGraph (strict)"("Y Scale.Scale Fit"=u8 2 ("Y Scale Fit")) -> ()  [unwired: 2 in, 2 out]
      }
      frame #2 {
        w546 = u16 1 items=["Single Values", "Curves", "Waveforms", "Multimeter"] ("Type")
        n209 = local read "Y-Resolution"() -> (w518:u8)
        n210 = case shown="\"Chinese\"" w519 {
          tunnel: ["L\u0000o\u0000w\u0000e\u0000r\u0000" ("Name") "\u000bN" ("Name")] -> w524
          tunnel: ["L\u0000i\u0000m\u0000i\u0000t\u0000" ("Name") "P–" ("Name")] -> w523
          tunnel: ["U\u0000p\u0000p\u0000e\u0000r\u0000" ("Name") "\nN" ("Name")] -> w525
          frame "English", Default {
          }
          frame "Chinese" {
          }
        }
        n211 = case shown="1" w533 {
          tunnel: w539 -> [w596 w598 w600]
          tunnel: [w595 w597 w599] -> w538
          frame 0, Default {
            n212 = Unbundle By Name(w596) -> ("X unit"=w595:string)
          }
          frame 1 {
            n213 = Unbundle By Name(w598) -> ("Y unit"=w597:string)
          }
          frame 2 {
            n214 = Unbundle By Name(w600) -> ("Z unit"=w599:string)
          }
        }
        n215 = local read "Tolerance"() -> (w548:u16)
        n216 = call "CRYConvert Unicode to ASCII.vi"("Unicode"=w523) -> ("ASCII"=w520:string)  [unwired: 4 in]
        n217 = local read "Step Name"() -> (w530:string)
        n218 = call "CRYConvert Unicode to ASCII.vi"("Unicode"=w524) -> ("ASCII"=w522:string)  [unwired: 4 in]
        n219 = call "CRYConvert Unicode to ASCII.vi"("Unicode"=w525) -> ("ASCII"=w521:string)  [unwired: 4 in]
        n220 = local read "Curve Name"() -> (w529:string)
        n221 = local read "Type"() -> (w551:u16)
        n222 = Equal?(x=u16 5, y=w548) -> (x = y?=w564:bool)
        n223 = Equal?(x=w548, y=u16 3) -> (x = y?=w563:bool)
        n224 = case shown="\"English\", Default" w519 {
          tunnel: [w581 w588] -> w554
          tunnel: [w580 w587] -> w553
          tunnel: w530 -> [w579 w586]
          tunnel: w522 -> [w577 w585]
          tunnel: w521 -> [w576 w584]
          tunnel: w520 -> [w575 w583]
          frame "Chinese" {
            w578 = " " ("Name")
            n225 = Concatenate Strings(w579, w578, w576, w575) -> (w581:string)
            n226 = Concatenate Strings(w579, w578, w577, w575) -> (w580:string)
          }
          frame "English", Default {
            w582 = " " ("Name")
            n227 = Concatenate Strings(w586, w582, w584, w582, w583) -> (w588:string)
            n228 = Concatenate Strings(w586, w582, w585, w582, w583) -> (w587:string)
          }
        }
        n229 = Not Equal?(x=w551, y=w546) -> (x != y?=w547:bool)
        n230 = Or(x=w564, y=w563) -> (x .or. y?=w561:bool)
        n231 = case shown="True" w547 {
          tunnel: [w680 w690] -> w527
          tunnel: [w677 w689] -> w556
          tunnel: w548 -> [w679 _]
          tunnel: w519 -> [w676 w688]
          tunnel: w518 -> [_ w683]
          frame False {
            n232 = case shown="\"Chinese\"" w676 {
              tunnel: ["T\u0000o\u0000l\u0000e\u0000r\u0000a\u0000n\u0000c\u0000e\u0000 \u0000c\u0000u\u0000r\u0000v\u0000e\u0000s\u0000" "FhP–" ("Unicode")] -> w680
              frame "English", Default {
              }
              frame "Chinese" {
              }
            }
            n233 = property on="Tolerance" class="Ring (strict)"() -> ("Strings []"=w678:string[])  [unwired: 2 in, 2 out]
            n234 = Index Array(array=w678, index=w679) -> (element=w677:string)
          }
          frame True {
            n235 = local read "min"() -> (w685:dbl)
            n236 = local read "Limits"() -> (w691:u16)
            n237 = local read "max"() -> (w687:dbl)
            n238 = call "CRYRepresent numeric by precission.vi"("Pprecision"=w683, "Numeric In"=w685) -> ("output string"=w684:string)  [unwired: 7 in, 2 out]
            n239 = call "CRYRepresent numeric by precission.vi"("Pprecision"=w683, "Numeric In"=w687) -> ("output string"=w686:string)  [unwired: 7 in, 2 out]
            n240 = case shown="\"Chinese\"" w688 {
              tunnel: w691 -> [w696 w710]
              tunnel: [w695 w709] -> w690
              tunnel: [w694 w708] -> w689
              tunnel: w686 -> [w693 w707]
              tunnel: w684 -> [w692 w706]
              frame "English", Default {
                n241 = case shown="2.." w696 {
                  tunnel: ["M\u0000a\u0000x\u0000i\u0000m\u0000u\u0000m\u0000" "M\u0000i\u0000n\u0000i\u0000m\u0000u\u0000m\u0000" "M\u0000a\u0000x\u0000/\u0000M\u0000i\u0000n\u0000"] -> w695
                  tunnel: [w697 w699 w704] -> w694
                  tunnel: w693 -> [w697 _ w702]
                  tunnel: w692 -> [_ w699 w701]
                  frame ..0 {
                  }
                  frame 1 {
                  }
                  frame 2.. {
                    n242 = Concatenate Strings(w702, "/", w701) -> (w704:string)
                  }
                }
              }
              frame "Chinese" {
                n243 = case shown="..0" w710 {
                  tunnel: ["\u0000g'Y<P" "\u0000g\u000f\\<P" "\u0000g'Y<P/\u0000\u0000g\u000f\\<P"] -> w709
                  tunnel: [w711 w713 w719] -> w708
                  tunnel: w707 -> [w711 _ w717]
                  tunnel: w706 -> [_ w713 w716]
                  frame ..0 {
                  }
                  frame 1 {
                  }
                  frame 2.. {
                    n244 = Concatenate Strings(w717, "/", w716) -> (w719:string)
                  }
                }
              }
            }
          }
        }
        n245 = case shown="True" w561 {
          tunnel: w536 -> [_ w729]
          tunnel: w567 -> [_ w733]
          tunnel: w568 -> [_ w732]
          tunnel: [w722 w731] -> w543
          tunnel: w563 -> [_ w725]
          tunnel: w519 -> [_ w723]
          frame False {
            n246 = call "CRYUnflatten Data.vi"() -> ("Datum"=w722:T5)  [unwired: 1 in, 10 out]
          }
          frame True {
            n247 = for {
              tunnel: w732 -> [w747] mode=indexing
              tunnel: [w745] -> w730 mode=indexing
              tunnel: w733 -> [w744] mode=indexing
              n248 = Unbundle By Name(w744) -> ("z"=w743:dbl)
              n249 = Unbundle(w747) -> ("Hz"=w746:dbl, "dB"=w742:dbl)
              n250 = Bundle("Hz"=w746, "dB"=w742, "z"=w743) -> (w745:cluster{"Hz":dbl, "dB":dbl, "z":dbl})  [unwired: 1 out]
            }
            n251 = case shown="\"English\", Default" w723 {
              tunnel: w725 -> [w735 w739]
              tunnel: [w734 w738] -> w726
              frame "English", Default {
                n252 = case shown="False" w735 {
                  tunnel: [" \u0000A\u0000l\u0000i\u0000g\u0000n\u0000e\u0000d\u0000" " \u0000F\u0000l\u0000o\u0000a\u0000t\u0000e\u0000d\u0000"] -> w734
                  frame False {
                  }
                  frame True {
                  }
                }
              }
              frame "Chinese" {
                n253 = case shown="True" w739 {
                  tunnel: ["s^ûy" ("Unicode") "nm¨R" ("Unicode")] -> w738
                  frame False {
                  }
                  frame True {
                  }
                }
              }
            }
            n254 = Unbundle By Name(w729) -> ("Name"=w728:string)
            n255 = call "CRYConvert Unicode to ASCII.vi"("Unicode"=w726) -> ("ASCII"=w724:string)  [unwired: 4 in]
            n256 = Concatenate Strings(w728, w724) -> (w727:string)
            n257 = Bundle By Name(cluster=w729, "Curve"=w730, "Name"=w727) -> (w731:T5)
          }
        }
        n258 = call "CRYResult name channel append.vi"("Curve selected"=w529, "Limit step name (no ext.)"=w554) -> ("Result name with channel suffix"=w555:string)  [unwired: 9 out]
        n259 = call "CRYResult name channel append.vi"("Curve selected"=w529, "Limit step name (no ext.)"=w553) -> ("Result name with channel suffix"=w535:string)  [unwired: 9 out]
        n260 = call "CRYResult name channel append.vi"("Curve selected"=w529, "Limit step name (no ext.)"=w530) -> ("Result name with channel suffix"=w528:string)  [unwired: 9 out]
        n261 = Equal?(x="deg", y=w538) -> (x = y?=w557:bool)
        n262 = for {
          tunnel: w574 -> [w763] mode=indexing
          tunnel: [w762] -> w573 mode=indexing
          tunnel: w557 -> [w761]
          n263 = case shown="True" w761 {
            tunnel: [w768 w773] -> w762
            tunnel: w763 -> [w765 w771]
            frame False {
              n264 = Unbundle(w765) -> ("Hz"=w767:dbl, "y"=w766:dbl)
              n265 = Bundle("Hz"=w767, "y"=w766, 0.0) -> (w768:cluster{"Hz":dbl, "y":dbl, dbl})  [unwired: 1 out]
            }
            frame True {
              n266 = Unbundle(w771) -> ("Hz"=w772:dbl, "y"=w770:dbl)
              n267 = Bundle("Hz"=w772, 0.0, "y"=w770) -> (w773:cluster{"Hz":dbl, dbl, "y":dbl})  [unwired: 1 out]
            }
          }
        }
        n268 = for {
          tunnel: w570 -> [w750] mode=indexing
          tunnel: [w749] -> w571 mode=indexing
          tunnel: w557 -> [w748]
          n269 = case shown="False" w748 {
            tunnel: [w755 w760] -> w749
            tunnel: w750 -> [w751 w758]
            frame False {
              n270 = Unbundle(w751) -> ("Hz"=w753:dbl, "y"=w752:dbl)
              n271 = Bundle("Hz"=w753, "y"=w752, 0.0) -> (w755:cluster{"Hz":dbl, "y":dbl, dbl})  [unwired: 1 out]
            }
            frame True {
              n272 = Unbundle(w758) -> ("Hz"=w759:dbl, "y"=w757:dbl)
              n273 = Bundle("Hz"=w759, 0.0, "y"=w757) -> (w760:cluster{"Hz":dbl, dbl, "y":dbl})  [unwired: 1 out]
            }
          }
        }
        n274 = Bundle By Name(cluster=w536, "Curve"=w573, "Name"=w555) -> (w572:T5)
        n275 = Bundle By Name(cluster=w536, "Curve"=w571, "Name"=w535) -> (w569:T5)
        n276 = call "CRYConvert Unicode to ASCII.vi"("Unicode"=w527) -> ("ASCII"=w526:string)  [unwired: 4 in]
        n277 = local read "Type"() -> (w534:u16)
        n278 = Not Equal?(x=w534, y=u16 2) -> (x != y?=w544:bool)
        n279 = case shown="..0" w552 {
          tunnel: ["dB" w721] -> w562
          tunnel: w538 -> [_ w721]
          frame ..0 {
          }
          frame 1.. {
          }
        }
        n280 = case shown="True" w544 {
          tunnel: w572 -> [w608 w634]
          tunnel: w569 -> [w607 w632]
          tunnel: w543 -> [_ w644]
          tunnel: w561 -> [w606 w643]
          tunnel: w560 -> [w603 w641]
          tunnel: [w601 w640] -> w559
          tunnel: w538 -> [w604 w638]
          tunnel: w552 -> [w605 w637]
          tunnel: "single val" -> [w602 w636]
          tunnel: w534 -> [_ w635]
          frame False {
            n281 = local read "Limits"() -> (w609:u16)
            n282 = case shown="False" w606 {
              tunnel: w607 -> [w614 w622]
              tunnel: [w613 w624] -> w610
              tunnel: w608 -> [w612 w623]
              tunnel: w609 -> [w611 _]
              frame False {
                n283 = case shown="..0" w611 {
                  tunnel: w612 -> [w616 _ w621]
                  tunnel: [w615 w618 w620] -> w613
                  tunnel: w614 -> [_ w617 w619]
                  frame ..0 {
                    n284 = Build Array(w616) -> (w615:T5[])
                  }
                  frame 1 {
                    n285 = Build Array(w617) -> (w618:T5[])
                  }
                  frame 2.. {
                    n286 = Build Array(w621, w619) -> (w620:T5[])
                  }
                }
              }
              frame True {
                n287 = Build Array(w623, w622) -> (w624:T5[])
              }
            }
            n288 = for {
              tunnel: [w625] -> w601 mode=indexing
              tunnel: w610 -> [w627] mode=indexing
              tunnel: w605 -> [w630]
              tunnel: w604 -> [w629]
              tunnel: w603 -> [w628]
              tunnel: w602 -> [w626]
              n289 = Bundle By Name(cluster=w627, "Y data"=w630, "Y unit"=w629, "Y dB ref"=w628, "single val"=w626) -> (w625:T5)
            }
          }
          frame True {
            n290 = case shown="0, Default" w635 {
              tunnel: w634 -> [w652 w654]
              tunnel: [w651 w654] -> w633
              tunnel: w632 -> [w650 w653]
              tunnel: [w649 w653] -> w631
              frame 0, Default {
                w646 = FALSE ("display X")
                w648 = FALSE ("display X")
                n291 = Bundle By Name(cluster=w652, "display X"=w646, "display Y"=TRUE, "display Z"=w646) -> (w651:T5)
                n292 = Bundle By Name(cluster=w650, "display X"=w648, "display Y"=TRUE, "display Z"=w648) -> (w649:T5)
              }
              frame 1 {
              }
            }
            n293 = local read "Limits"() -> (w639:u16)
            n294 = case shown="True" w643 {
              tunnel: w644 -> [_ w673]
              tunnel: w631 -> [w664 w672]
              tunnel: [w663 w675] -> w642
              tunnel: w633 -> [w662 w674]
              tunnel: w639 -> [w661 _]
              frame False {
                n295 = case shown="2.." w661 {
                  tunnel: w662 -> [w666 _ w671]
                  tunnel: [w665 w668 w670] -> w663
                  tunnel: w664 -> [_ w667 w669]
                  frame ..0 {
                    n296 = Build Array(w666) -> (w665:T5[])
                  }
                  frame 1 {
                    n297 = Build Array(w667) -> (w668:T5[])
                  }
                  frame 2.. {
                    n298 = Build Array(w671, w669) -> (w670:T5[])
                  }
                }
              }
              frame True {
                n299 = Build Array(w674, w673, w672) -> (w675:T5[])
              }
            }
            n300 = for {
              tunnel: [w655] -> w640 mode=indexing
              tunnel: w642 -> [w657] mode=indexing
              tunnel: w637 -> [w660]
              tunnel: w638 -> [w659]
              tunnel: w641 -> [w658]
              tunnel: w636 -> [w656]
              n301 = Bundle By Name(cluster=w657, "Y data"=w660, "Y unit"=w659, "Y dB ref"=w658, "single val"=w656) -> (w655:T5)
            }
          }
        }
        n302 = call "CRYUnflatten Results.vi"() -> ("Result"=w540:T2)  [unwired: 1 in, 10 out]
        n303 = call "CRYRepresent numeric by precission.vi"("Pprecision"=w518, "Numeric In"=w532) -> ("Numeric Out"=w531:dbl)  [unwired: 7 in, 2 out]
        n304 = Bundle By Name(cluster=w540, "Name"=w528, "Margin"=w531, "unit"=w562, "Verdict"=w537, "Limit"=w526, "Max/Min"=w556) -> (w549:T2)
        n305 = call "CRYDAT to Waveform.vi"("Curve In"=w543) -> ("Waveform Out"=w542:T3)  [unwired: 1 in, 9 out]
        n306 = Build Array(w542) -> (w541:T3[])
      }
    }
    n307 = Build Array (concatenate)(w129, w131) -> (w130:T4)
    n308 = Build Array (concatenate)(w125, w124) -> (w126:T3[])
  }
  "Data Out" <- w37
  "Waveforms Out" <- w39
  "Results Out" <- w33
  n309 = local read "magn/phase"() -> (w35:u16)
  n310 = Index Array(array=w33, index=0) -> (element=w36:T2)
  n311 = case shown="2" w28 {
    tunnel: w37 -> [w778 w791 w813]
    tunnel: w39 -> [_ _ w812]
    tunnel: w35 -> [_ w790 _]
    tunnel: w2 -> [w777 w786 w811]
    tunnel: [w776 w784 w809] -> w17
    tunnel: [w775 w785 w809] -> w18
    tunnel: [w774 w783 w810] -> w15
    tunnel: T5[] [] -> [w775 w784 w809]
    tunnel: T3[] [] -> [w774 w783 _]
    frame 0, Default {
      n312 = for {
        tunnel: w778 -> [w782] mode=indexing
        tunnel: [w780] -> w776 mode=indexing
        tunnel: w777 -> [w781]
        n313 = Bundle By Name(cluster=w782, "protected"=FALSE, "Step No."=w781) -> (w780:T5)
      }
    }
    frame 1 {
      n314 = case shown="2" w790 {
        tunnel: [w805 w807] -> w787
        tunnel: [w805 FALSE ("display X")] -> w788
        tunnel: [FALSE ("display X") w807] -> w789
        frame 0, 1, Default {
          w805 = TRUE ("display X")
        }
        frame 2 {
          w807 = TRUE ("display X")
        }
      }
      n315 = for {
        tunnel: w791 -> [w795] mode=indexing
        tunnel: [w793] -> w785 mode=indexing
        tunnel: w787 -> [w803]
        tunnel: w788 -> [w802]
        tunnel: w789 -> [w801]
        tunnel: w786 -> [w800]
        n316 = call "CRYGet Resolution_Steps of Curves.vi"("Curve In"=w795) -> ("Steps Out"=w796:i32, "Original Resolution Out"=w797:string)  [unwired: 9 in]
        n317 = Bundle By Name(cluster=cluster{"Original Res":string, "Steps":i32} {"Original Res"="", "Steps"=0} ("unflattened test info data"), "Original Res"=w797, "Steps"=w796) -> (w798:cluster{"Original Res":string, "Steps":i32})
        n318 = call "CRYFlatten Curve Test Info.vi"("unflattened test info data"=w798) -> ("Flattened Data"=w794:string)  [unwired: 10 in]
        n319 = Bundle By Name(cluster=w795, "protected"=FALSE, "Step No."=w800, "display X"=w803, "display Y"=w802, "display Z"=w801, "Test Info"=w794) -> (w793:T5)
      }
    }
    frame 2 {
      n320 = local read "Tolerance"() -> (w808:u16)
      n321 = Equal?(x=w808, y=u16 3) -> (x = y?=w818:bool)
      n322 = Equal?(x=w808, y=u16 5) -> (x = y?=w817:bool)
      n323 = Or(x=w818, y=w817) -> (x .or. y?=w814:bool)
      n324 = case shown="True" w814 {
        tunnel: w813 -> [w821 w835]
        tunnel: w812 -> [_ w837]
        tunnel: w811 -> [w820 w831]
        tunnel: [w819 w830] -> w810
        frame False {
          n325 = for {
            tunnel: w821 -> [w827] mode=indexing
            tunnel: [w823] -> w819 mode=indexing
            tunnel: w820 -> [w824]
            w825 = TRUE ("display X")
            n326 = Bundle By Name(cluster=w827, "protected"=FALSE, "Step No."=w824, "display X"=w825, "display Y"=w825) -> (w826:T5)
            n327 = call "CRYDAT to Waveform.vi"("Curve In"=w826) -> ("Waveform Out"=w823:T3)  [unwired: 1 in, 9 out]
          }
        }
        frame True {
          w833 = TRUE ("display Y")
          n328 = for {
            tunnel: w835 -> [w843] mode=indexing
            tunnel: [w839] -> w832 mode=indexing
            tunnel: w831 -> [w840]
            w841 = TRUE ("display X")
            n329 = Bundle By Name(cluster=w843, "protected"=FALSE, "Step No."=w840, "display X"=w841, "display Y"=w841) -> (w842:T5)
            n330 = call "CRYDAT to Waveform.vi"("Curve In"=w842) -> ("Waveform Out"=w839:T3)  [unwired: 1 in, 9 out]
          }
          n331 = Index Array(array=w837, index=0) -> (element=w834:T3)
          n332 = Bundle By Name(cluster=w834, "protected"=FALSE, "Step No."=w831, "display Y"=w833, "display X"=w833) -> (w829:T3)
          n333 = Build Array (concatenate)(w829, w832) -> (w830:T3[])
        }
      }
    }
  }
  n334 = Bundle By Name(cluster=w36, "Step No."=w2) -> (w26:T2)
  n335 = Build Array(w26) -> (w16:T2[])
  n336 = case shown="True" w32 {
    tunnel: w33 -> [_ w846]
    frame False {
    }
    frame True {
      n337 = while {
        tunnel: w846 -> [_]
        tunnel: [w848] -> w845
        stop <- w848 stop-if-true
        n338 = event shown="[2] Key Down" {
          selector: _ -> [_ _ _]
          dyn-events: _ -> [_ _ _]
          timeout: 10 -> [_ _ _]
          event Timeout {
            n339 = event-data() -> ()  [unwired: 3 out]
          }
          event Panel Close? {
            n340 = event-data() -> ()  [unwired: 5 out]
            n341 = local write "stop"(TRUE ("stop")) -> ()
            n342 = event-data("Discard?"=TRUE) -> ()  [unwired: 1 in, 1 out]
          }
          event Key Down {
            n343 = event-data() -> ("VKey"=w856:T15)  [unwired: 7 out]
            n344 = Equal?(x=w856, y=eventvkey."Return") -> (x = y?=w857:bool)
            n345 = Equal?(x=w856, y=eventvkey."Enter") -> (x = y?=w858:bool)
            n346 = Or(x=w858, y=w857) -> (x .or. y?=w855:bool)
            n347 = local write "stop"(w855) -> ()
          }
        }
        n348 = global read "CRYProject Run Control Global.vi" "Cont Seq"() -> (w852:bool)
        n349 = global read "CRYProject Run Control Global.vi" "Aborted"() -> (w850:bool)
        n350 = global read "CRYMainGlobal.vi" "STOP"() -> (w849:bool)
        n351 = Compound Arithmetic op=OR(w849, w850, w852, "stop") -> (w848:bool)
      }
      n352 = Not(x=w845) -> (.not. x?=w844:bool)
      n353 = property class="VI"("Front Panel.Open"=w844) -> ()  [unwired: 2 in, 2 out]
    }
  }
  n354 = Index Array(array=w20, index=1) -> (element=w14:bool)
  n355 = global read "CRYProject Run Control Global.vi" "RunState"() -> (w11:bool)
  n356 = Select(t="Overwrite" ("Y unit"), s=w14, f="Repeat") -> (s? t:f=w19:string)
  n357 = case shown="True" w11 {
    tunnel: ["Apply" ("sOption1") "Run" ("Type In")] -> w10
    tunnel: ["APPLY_CURVE" ("Type In") "RUN_CURVE" ("Type In")] -> w9
    frame False {
    }
    frame True {
    }
  }
  n358 = case shown="True" w14 {
    tunnel: w18 -> [w874 w878]
    tunnel: w17 -> [w873 w877]
    tunnel: w16 -> [w872 w876]
    tunnel: w15 -> [w871 w875]
    tunnel: [w870 w878] -> w6
    tunnel: [w869 w877] -> w5
    tunnel: [w868 w876] -> w4
    tunnel: [w867 w875] -> w3
    tunnel: w13 -> [w866 _]
    tunnel: w9 -> [w865 _]
    frame False {
      n359 = call "CRYPrefix Curve Name.vi"("Type In"=w865, "Curves In"=w874, "Values In"=w873, "Results In"=w872, "Waves In"=w871, "Repeat State Array In"=w866) -> ("Curves Out"=w870:T4, "Values Out"=w869:T4, "Results Out"=w868:T16, "Waves Out"=w867:T10)  [unwired: 6 in]
    }
    frame True {
    }
  }
  n360 = call "CRYInsert Socket.vi"("sOption2"=w19, "Step No."=w2, "sOption1"=w10, "Waves"=w3, "Results"=w4, "Values"=w5, "Curves"=w6) -> ("Inserted Names Out"=→"Inserted Names Out":string[])  [unwired: 4 in]
  n361 = call "CRYGet Type from Data.vi"("Waves"=w3, "Results"=w4, "Values"=w5, "Curves"=w6) -> ("Type"=→"Types Out":string[])  [unwired: 7 in]
